vi "LSX Get Hdi Speed Index Single Axis.vi"(8 "error in (no error)":errorcluster, 9 "plIndex":i32, 10 "lAxis":i32, 11 "lLSID":i32) -> (0 "error out":errorcluster, 1 "plIndex out":i32, 3 "function return":i32)   [LabVIEW 2018, in "Tango.lvlib"]
doc: "TANGOAPI int TANGOCALL LSX_GetHdiSpeedIndexSingleAxis (int lLSID, int lAxis, int *plIndex);"
uses:
  Tango.lvlib
  SubVIs/Tango_DLL.dll
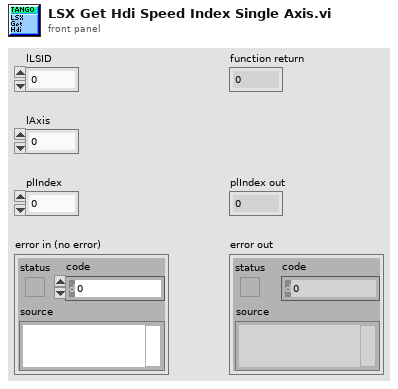
[diagram p1: front panel]
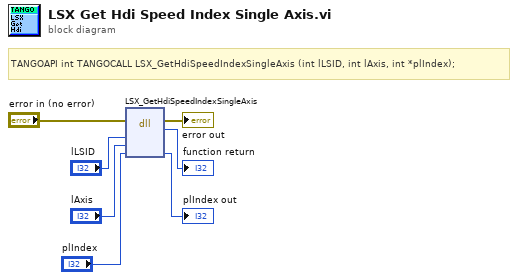
[diagram p0: block diagram]
diagram:
  # "TANGOAPI int TANGOCALL LSX_GetHdiSpeedIndexSingleAxis (int lLSID, int lAxis, int *plIndex);"
  n1 = dll-call lib="C:/Users/Familie/Documents/LabviewIX81/lib/TANGO Stage/SubVIs/Tango_DLL.*" fn="LSX_GetHdiSpeedIndexSingleAxis"(error in="error in (no error)", "lLSID"="lLSID", "lAxis"="lAxis", "plIndex"="plIndex") -> (error out=→"error out":errorcluster, →"function return":i32, "plIndex"=→"plIndex out":i32)  [unwired: 4 in, 1 out]
